vi "Initialize Alias Endpoint Strings.vi"(8 "error in (no error)":errorcluster, 10 "Endpoints":T1, 11 "Aliases Ctl Ref":refnum<vi>) -> (0 "error out":errorcluster, 3 "Aliases Ctl Ref out":refnum<vi>)   [LabVIEW 2017, in "Routing and Faulting System Explorer.lvlib"]
uses:
  Routing and Faulting System Explorer.lvlib
  <vilib>/Utility/miscctls.llb/LVComboBoxStrsAndValuesArrayTypeDef.ctl
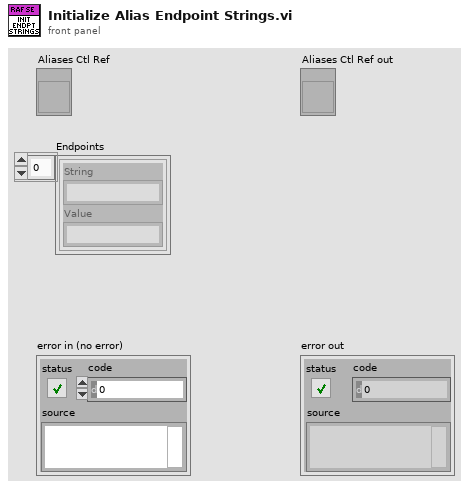
[diagram p1: front panel]
types:
  T1 = typedef "LVComboBoxStrsAndValuesArrayTypeDef.ctl" = cluster{"String":string, "Value":string}[]
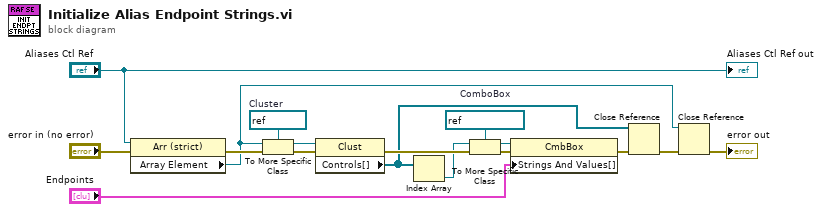
[diagram p0: block diagram]
diagram:
  w11 = refnum<vi> refnum  # ComboBox
  w14 = refnum<vi> refnum  # Cluster
  n1 = property class="Arr (strict)"(reference="Aliases Ctl Ref", error in="error in (no error)") -> (error out=w15:errorcluster, "Array Element"=w3:refnum<vi>)  [unwired: 1 out]
  n2 = To More Specific Class(target class=w14, reference=w3, error in=w15) -> (specific class reference=w12:refnum<vi>, error out=w13:errorcluster)
  n3 = property class="Clust"(reference=w12, error in=w13) -> (error out=w10:errorcluster, "Controls[]"=w5:refnum<vi>[])  [unwired: 1 out]
  n4 = Index Array(array=w5) -> (element=w7:refnum<vi>)  [unwired: 1 in]
  n5 = To More Specific Class(target class=w11, reference=w7, error in=w10) -> (specific class reference=w8:refnum<vi>, error out=w9:errorcluster)
  n6 = property class="CmbBox"(reference=w8, error in=w9, "Strings And Values[]"="Endpoints") -> (error out=w6:errorcluster)  [unwired: 1 out]
  n7 = Close Reference(reference=w5, error in (no error)=w6) -> (error out=w4:errorcluster)
  n8 = Close Reference(reference=w3, error in (no error)=w4) -> (error out=→"error out":errorcluster)
  "Aliases Ctl Ref out" <- "Aliases Ctl Ref"
